vi "U2000_USB_PM_OPC.vi"(7 "OPC Type [*OPC]":enum16{"*OPC", "*STB?"}(ring), 8 "error in (no error)":errorcluster, 9 "Maximum Time (10000ms)":u32=10000, 10 "Wait (100ms)":u32=100, 11 "VISA resource name":refnum<visa-resource-name>) -> (0 "error out":errorcluster, 3 "VISA resource name out":refnum<visa-resource-name>)   [LabVIEW 2015]
doc: "Waits for the current operation to finish. This VI should be called after Initiate VI.\n\n<B>Note:</B> \n\nUse this VI only with other low-level VIs. The high-level VIs automatically incorporate this functionality. This VI does not check the instrument status."
panel:
  out "Error":string="\n"
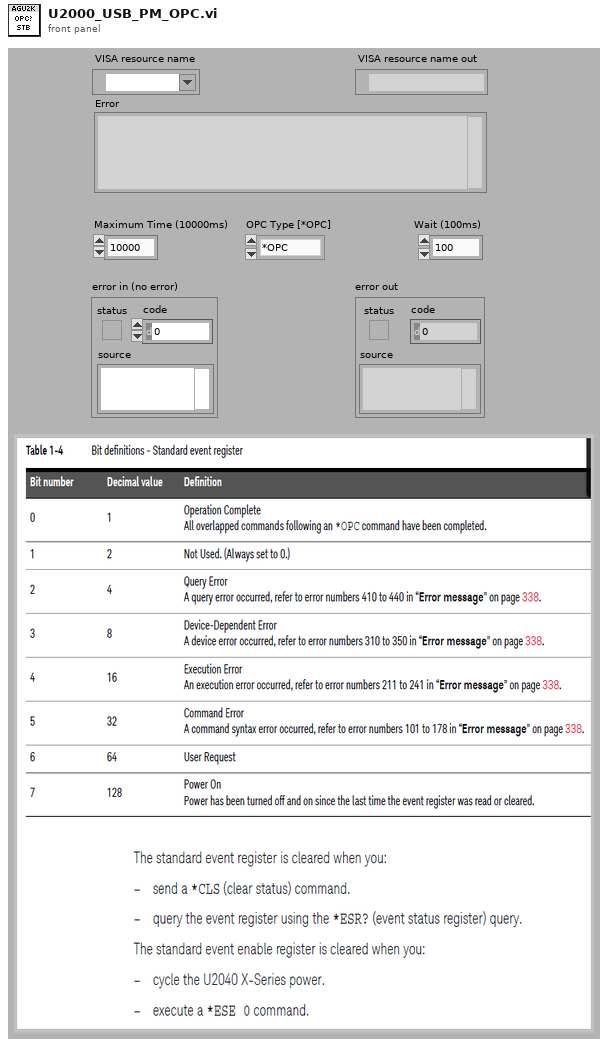
[diagram p1: front panel]
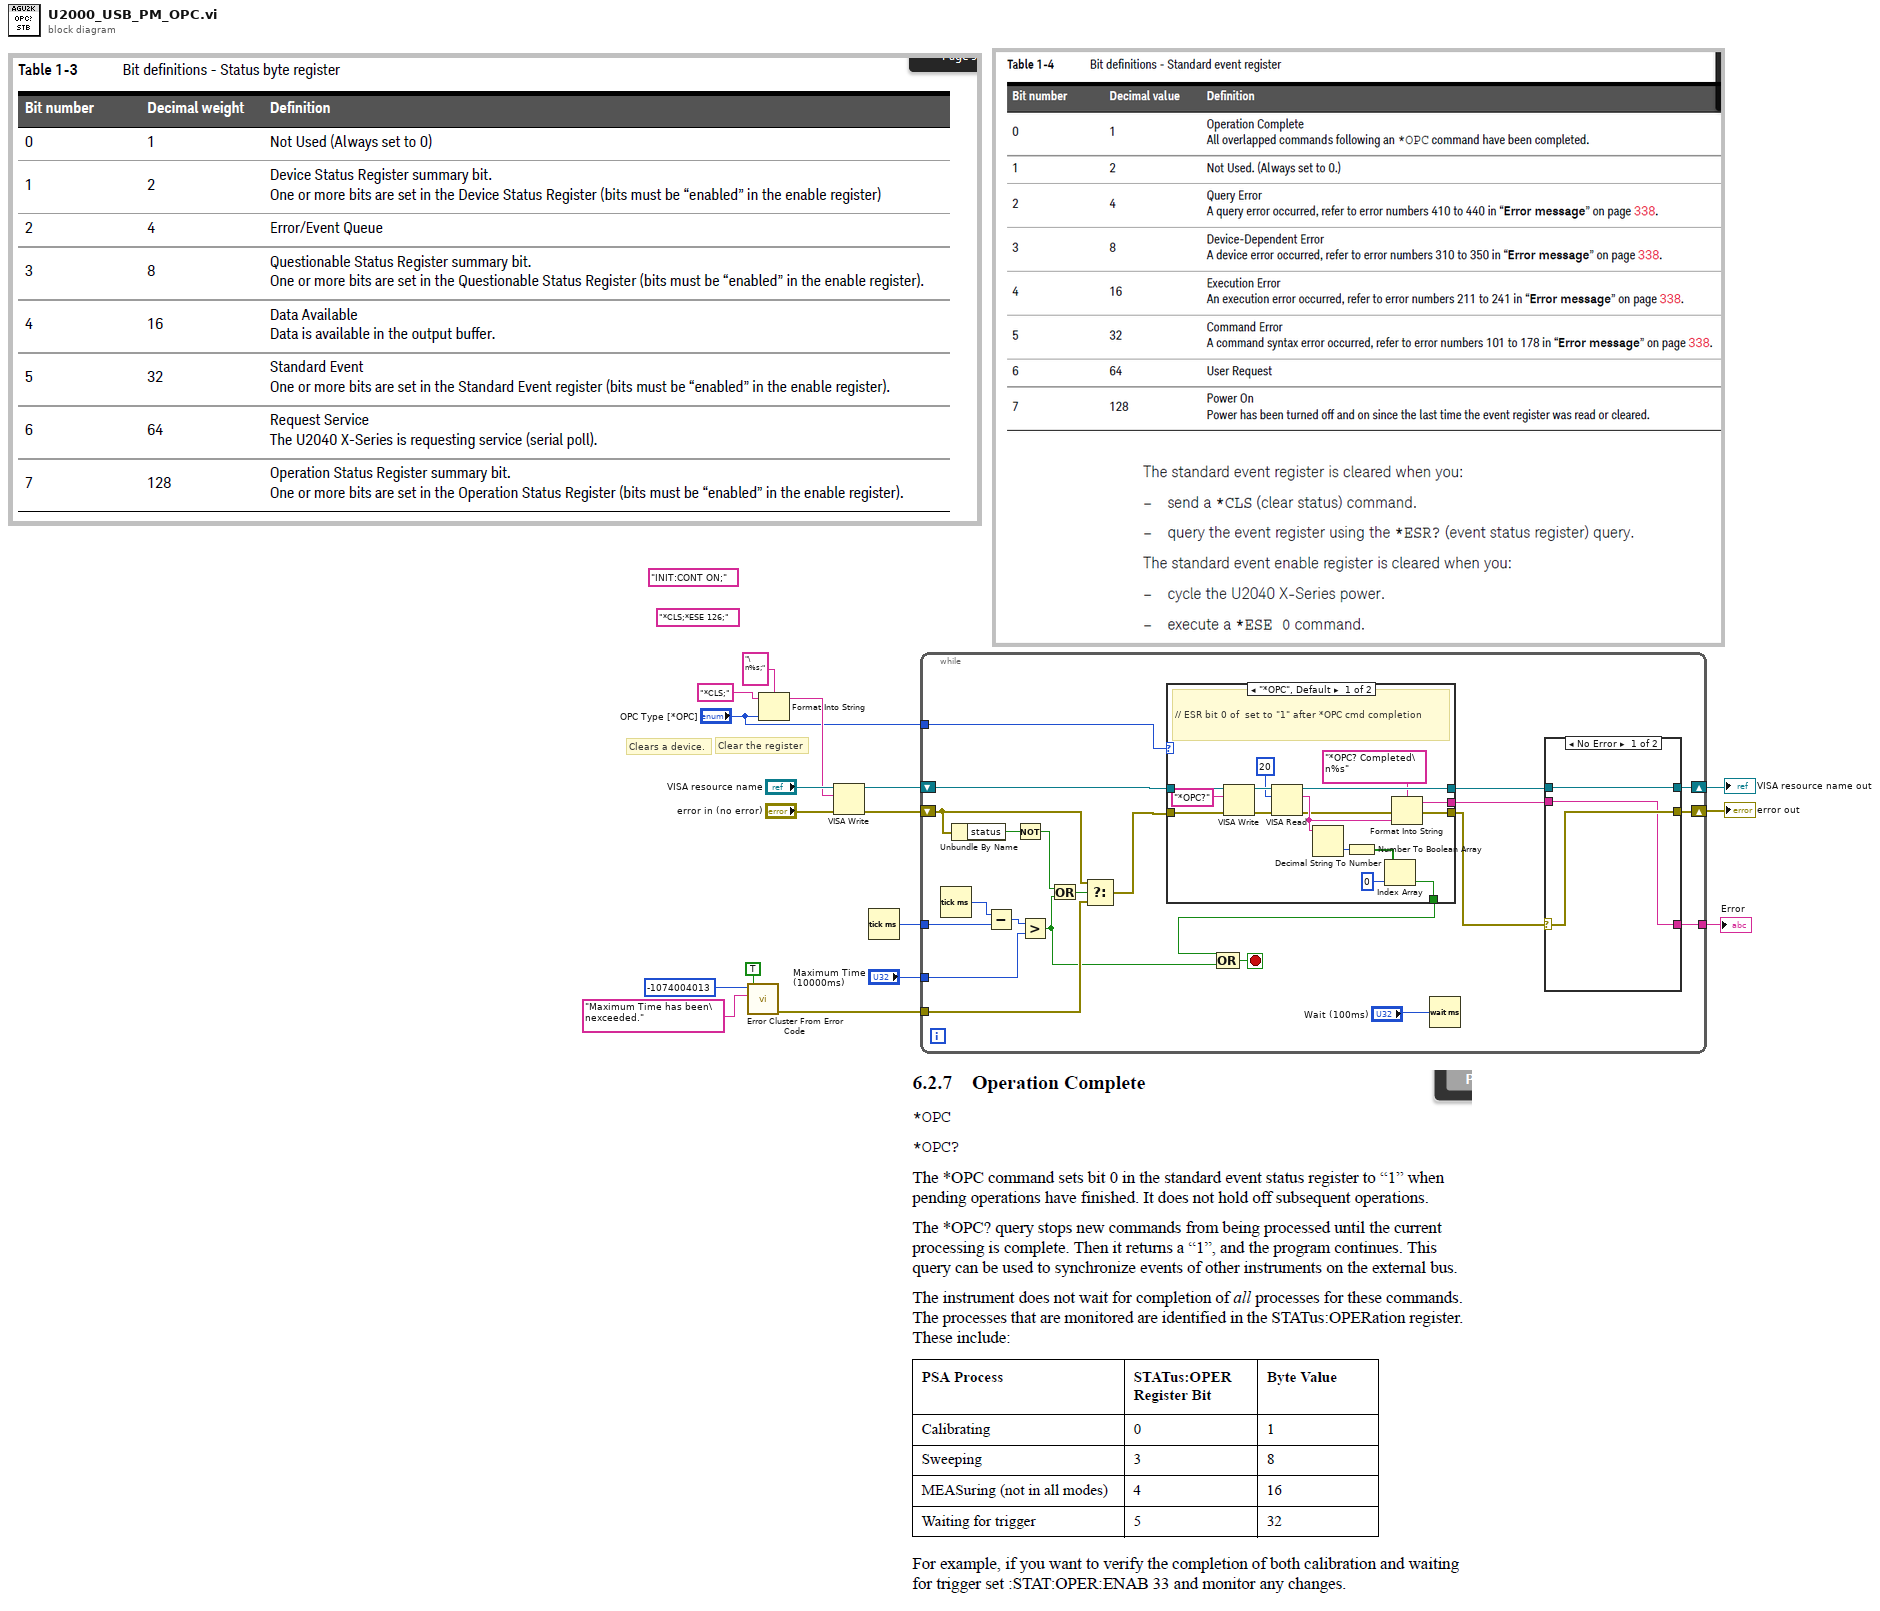
[diagram p0: block diagram]
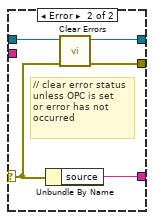
[diagram p2: hidden frame]
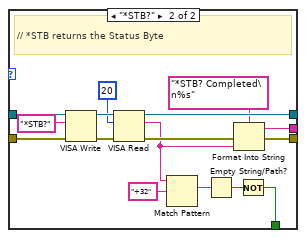
[diagram p3: hidden frame]
diagram:
  (unwired) "*CLS;*ESE 126;" ("write buffer")
  (unwired) "INIT:CONT ON;" ("write buffer")
  # "Clears a device."
  # "Clear the register"
  n1 = call <vilib>:"Error Cluster From Error Code.vi"("show call chain? (False)"=TRUE, "error message (\"\")"="Maximum Time has been\nexceeded." ("error message (\"\")"), "error code (0)"=-1074004013) -> ("error out"=w12:errorcluster)  [unwired: 6 in]
  n2 = Format Into String(format string="\n%s;", initial string="*CLS;" ("write buffer"), "OPC Type [*OPC]") -> (resulting string=w4:string)  [unwired: 1 in, 1 out]
  n3 = VISA Write(VISA resource name="VISA resource name", write buffer=w4, error in (no error)="error in (no error)") -> (VISA resource name out=w9:refnum<visa-resource-name>, error out=w8:errorcluster)  [unwired: 1 out]
  n4 = Tick Count (ms)() -> (millisecond timer value=w16:u32)
  n5 = while {
    tunnel: "Maximum Time (10000ms)" -> [w32]
    tunnel: w16 -> [w38]
    tunnel: w12 -> [w35]
    shift-right: [w24] -> w10
    shift-left: w8 -> [w34]
    shift-right: [w25] -> w11
    shift-left: w9 -> [w29]
    tunnel: "OPC Type [*OPC]" -> [w28]
    tunnel: [w20] -> w2
    stop <- w37 stop-if-true
    n6 = Tick Count (ms)() -> (millisecond timer value=w39:u32)
    n7 = Unbundle By Name(w34) -> ("status"=w31:bool)
    n8 = Subtract(x=w39, y=w38) -> (x-y=w33:u32)
    n9 = Not(x=w31) -> (.not. x?=w18:bool)
    n10 = Greater?(x=w33, y=w32) -> (0:w21:bool)
    n11 = Or(x=w18, y=w21) -> (x .or. y?=w36:bool)
    n12 = Select(t=w34, s=w36, f=w35) -> (s? t:f=w23:errorcluster)
    n13 = case shown="\"*OPC\", Default" w28 {
      tunnel: [w62 w78] -> w27
      tunnel: w23 -> [w59 w75]
      tunnel: w29 -> [w61 w77]
      tunnel: [w55 w64] -> w30
      tunnel: [w50 w71] -> w22
      tunnel: [w48 w69] -> w26
      frame "*OPC", Default {
        # "// ESR bit 0 of  set to \"1\" after *OPC cmd completion"
        n14 = VISA Write(VISA resource name=w61, write buffer="*OPC?", error in (no error)=w59) -> (VISA resource name out=w60:refnum<visa-resource-name>, error out=w58:errorcluster)  [unwired: 1 out]
        n15 = VISA Read(VISA resource name=w60, byte count=u32 20, error in (no error)=w58) -> (VISA resource name out=w62:refnum<visa-resource-name>, read buffer=w52:string, error out=w49:errorcluster)  [unwired: 1 out]
        n16 = Decimal String To Number(string=w52) -> (number=w53:i32)  [unwired: 2 in, 1 out]
        n17 = Number To Boolean Array(number=w53) -> (Boolean array=w56:bool[])
        n18 = Index Array(array=w56, index=0) -> (element=w55:bool)
        n19 = Format Into String(format string="*OPC? Completed\n%s" ("string"), error in=w49, w52) -> (resulting string=w48:string, error out=w50:errorcluster)  [unwired: 1 in]
      }
      frame "*STB?" {
        # "// *STB returns the Status Byte"
        n20 = VISA Write(VISA resource name=w77, write buffer="*STB?", error in (no error)=w75) -> (VISA resource name out=w76:refnum<visa-resource-name>, error out=w74:errorcluster)  [unwired: 1 out]
        n21 = VISA Read(VISA resource name=w76, byte count=u32 20, error in (no error)=w74) -> (VISA resource name out=w78:refnum<visa-resource-name>, read buffer=w65:string, error out=w70:errorcluster)  [unwired: 1 out]
        n22 = Match Pattern(string=w65, regular expression="+32") -> (match substring=w67:string)  [unwired: 1 in, 3 out]
        n23 = Empty String/Path?(string/path=w67) -> (empty?=w68:bool)
        n24 = Format Into String(format string="*STB? Completed\n%s" ("string"), error in=w70, w65) -> (resulting string=w69:string, error out=w71:errorcluster)  [unwired: 1 in]
        n25 = Not(x=w68) -> (.not. x?=w64:bool)
      }
    }
    n26 = Compound Arithmetic op=OR(w30, w21) -> (w37:bool)
    n27 = Wait (ms)(milliseconds to wait="Wait (100ms)") -> ()  [unwired: 1 out]
    n28 = case shown="No Error" w22 {
      selector: w22 -> [w41 w43]
      tunnel: w27 -> [w42 w46]
      tunnel: [w42 w46] -> w25
      tunnel: [w41 w45] -> w24
      tunnel: [w40 w44] -> w20
      tunnel: w26 -> [w40 _]
      frame No Error {
      }
      frame Error {
        # "// clear error status\nunless OPC is set\nor error has not\noccurred"
        n29 = Unbundle By Name(w43) -> ("source"=w44:string)
        n30 = call <vilib>:"Clear Errors.vi"("error in (no error)"=w43) -> ("error out"=w45:errorcluster)  [unwired: 5 in, 1 out]
      }
    }
  }
  "error out" <- w10
  "VISA resource name out" <- w11
  "Error" <- w2
